vi "Handle State Value Table Change.vi"(7 "Routing Channel Page Controls":T1, 8 "error in (no error)":errorcluster, 9 "OldVal":T3[](array[typedef]), 10 "NewVal":T3[](array[typedef]), 11 "routing channel in":T2 format="%.0x") -> (0 "error out":errorcluster, 3 "routing channel out":T2 format="%.0x")   [LabVIEW 2017, in "Routing and Faulting System Explorer.lvlib"]
uses:
  <vilib>/NI Veristand/Custom Device API/Custom Device Item Ref.ctl
  State-Value Row.ctl
  Routing Channel Page Controls.ctl
  88e8a73d-5bf6-438f-825b-ec6305f3fa8d.vi
  Routing and Faulting System Explorer.lvlib
  Scripting/Routing and Faulting Scripting.lvlib
  <vilib>/NI Veristand/Custom Device API/Custom Device API.lvlib
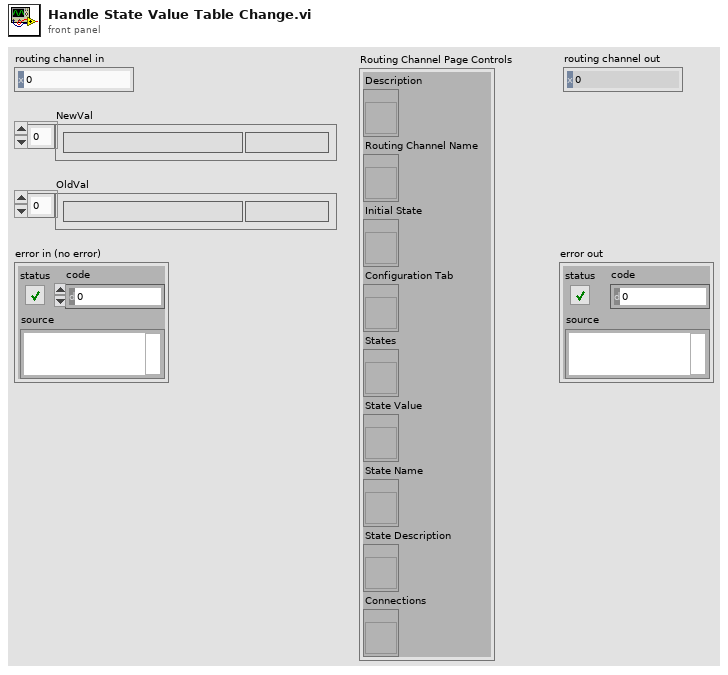
[diagram p1: front panel]
types:
  T1 = typedef "Routing and Faulting System Explorer.lvlib/Routing Channel Page Controls.ctl" = cluster{"Description":refnum<vi>, "Routing Channel Name":refnum<vi>, "Initial State":refnum<vi>, "Configuration Tab":refnum<vi>, "States":refnum<vi>, "State Value":refnum<vi>, "State Name":refnum<vi>, "State Description":refnum<vi>, "Connections":refnum<vi>}
  T2 = typedef "Custom Device API.lvlib/Custom Device Item Ref.ctl" = u64
  T3 = typedef "Routing and Faulting System Explorer.lvlib/State-Value Row.ctl" = cluster{"State":string, "State Value":string}
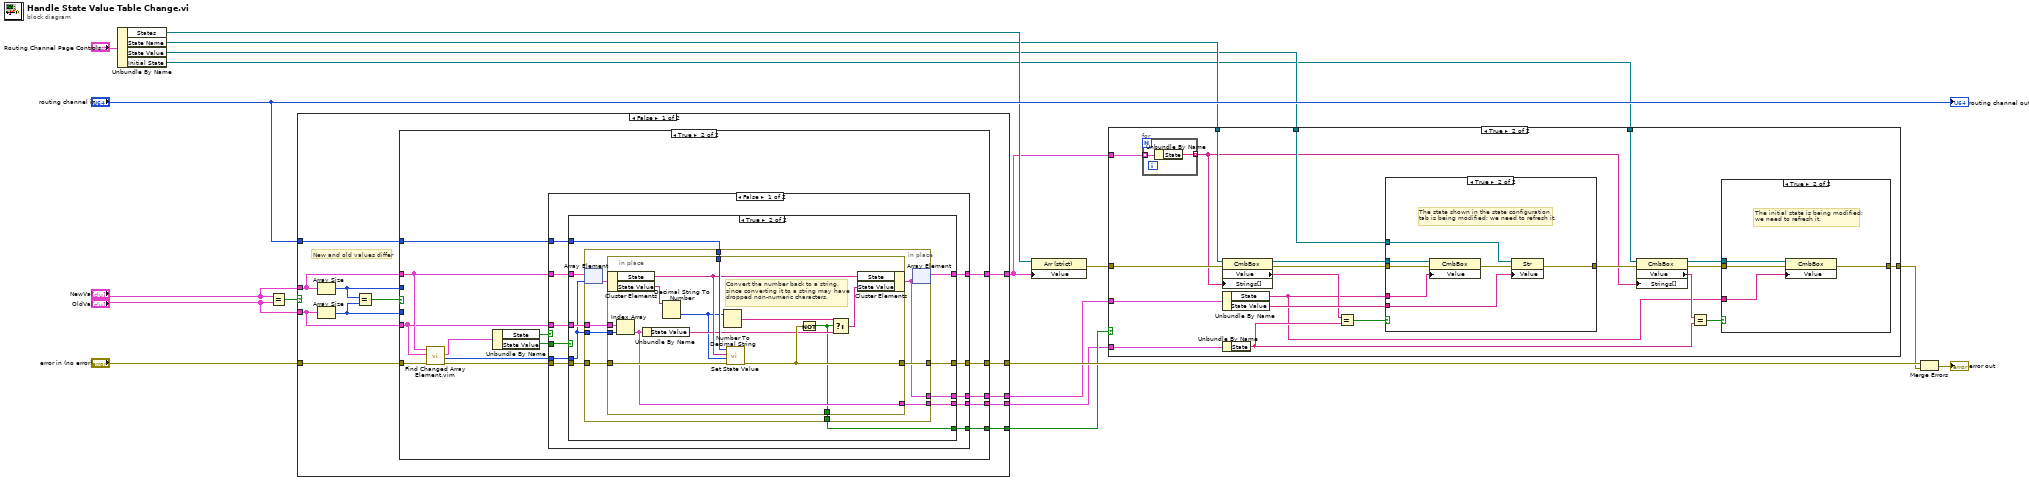
[diagram p0: block diagram]
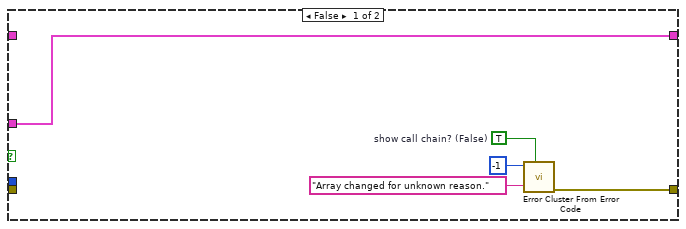
[diagram p3: hidden frame]
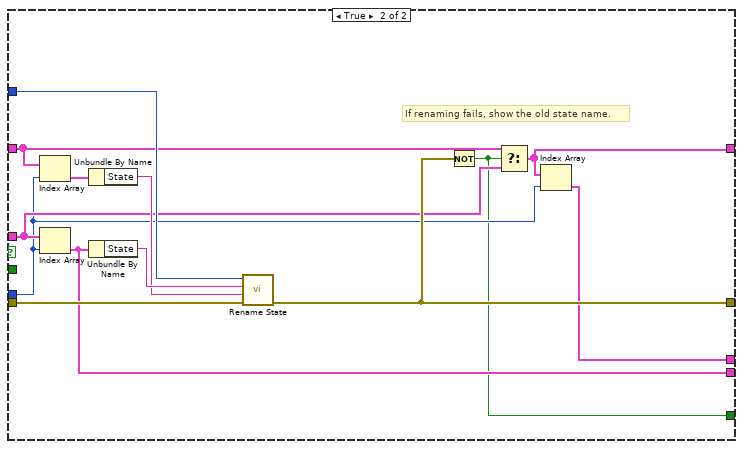
[diagram p4: hidden frame]
diagram:
  n1 = Unbundle By Name("Routing Channel Page Controls") -> ("States"=w10:refnum<vi>, "State Name"=w8:refnum<vi>, "State Value"=w4:refnum<vi>, "Initial State"=w1:refnum<vi>)
  n2 = Equal?(x="NewVal", y="OldVal") -> (x = y?=w13:bool)
  n3 = case shown="False" w13 {
    tunnel: "NewVal" -> [w27 w108]
    tunnel: "OldVal" -> [w26 _]
    tunnel: "routing channel in" -> [w25 _]
    tunnel: [w24 w109] -> w18
    tunnel: "error in (no error)" -> [w23 w109]
    tunnel: [w22 w108] -> w2
    tunnel: [w21 _] -> w7
    tunnel: [w20 _] -> w6
    tunnel: [w19 _] -> w5
    frame False {
      # "New and old values differ"
      n4 = Array Size(array=w27) -> (size(s)=w29:i32)
      n5 = Array Size(array=w26) -> (size(s)=w28:i32)
      n6 = Equal?(x=w29, y=w28) -> (x = y?=w30:bool)
      n7 = case shown="True" w30 {
        tunnel: w29 -> [_ _]
        tunnel: w28 -> [_ _]
        tunnel: w27 -> [_ w42]
        tunnel: w26 -> [w31 w37]
        tunnel: w25 -> [_ w44]
        tunnel: [w32 w41] -> w24
        tunnel: w23 -> [w32 w40]
        tunnel: [w31 w38] -> w22
        tunnel: [_ w35] -> w19
        tunnel: [_ w34] -> w20
        tunnel: [_ w33] -> w21
        frame False {
          # "This case can happen if items are inserted or removed from the array\nshortcut menu during runtime. This is a lot of extra code to handle,\nso the shortcut menu for the array on Endpoint Aliases Page.vi is\ncurrently disabled to prevent this code path.\nIf the shortcut menu is ever re-enabled, code for handling add/remove\nshould go in this case."
        }
        frame True {
          n8 = call "Find Changed Array Element.vim"("error in (no error)"=w40, "OldVal"=w37, "NewVal"=w42) -> ("error out"=w43:errorcluster, "Array Index"=w36:i32, "Element Changed"=w46:cluster{"State":bool, "State Value":bool})  [unwired: 6 in]
          n9 = Unbundle By Name(w46) -> ("State"=w45:bool, "State Value"=w39:bool)
          n10 = case shown="False" w45 {
            tunnel: w44 -> [w57 w107]
            tunnel: w43 -> [w54 w106]
            tunnel: w42 -> [w53 w101]
            tunnel: w37 -> [w50 w99]
            tunnel: [w55 w102] -> w41
            tunnel: w36 -> [w52 w97]
            tunnel: w39 -> [w56 _]
            tunnel: [w51 w100] -> w38
            tunnel: [w48 w98] -> w34
            tunnel: [w49 w96] -> w35
            tunnel: [w47 w95] -> w33
            frame False {
              n11 = case shown="True" w56 {
                tunnel: w57 -> [_ w70]
                tunnel: [w62 w71] -> w55
                tunnel: w54 -> [_ w72]
                tunnel: w53 -> [_ w69]
                tunnel: w52 -> [_ w66]
                tunnel: [w58 w68] -> w51
                tunnel: w50 -> [w58 w67]
                tunnel: [_ w65] -> w49
                tunnel: [_ w64] -> w48
                tunnel: [_ w63] -> w47
                frame False {
                  w59 = TRUE  # show call chain? (False)
                  n12 = call <vilib>:"Error Cluster From Error Code.vi"("show call chain? (False)"=w59, "error message (\"\")"="Array changed for unknown reason." ("error message (\"\")"), "error code (0)"=-1) -> ("error out"=w62:errorcluster)  [unwired: 6 in]
                }
                frame True {
                  n13 = in-place {
                    in-place-border: w72 -> [w81]
                    in-place-border: [w80] -> w71
                    in-place-border: w70 -> [w79]
                    in-place-border: w67 -> [w77]
                    in-place-border: w66 -> [w76]
                    in-place-border: [w75] -> w65
                    in-place-border: [w74] -> w64
                    in-place-border: [w73] -> w63
                    n14 = in-place-array #1(w69, w66) -> (w78:T3)
                    n15 = in-place {
                      in-place-border: w81 -> [w94]
                      in-place-border: [w93] -> w80
                      in-place-border: w79 -> [w92]
                      in-place-border: w77 -> [w88]
                      in-place-border: w76 -> [w87]
                      in-place-border: [w83] -> w74
                      in-place-border: [w82] -> w73
                      # "Convert the number back to a string,\nsince converting it to a string may have\ndropped non-numeric characters."
                      n16 = in-place-cluster #2(w78) -> ("State"=w89:string, "State Value"=w91:string)
                      n17 = Index Array(array=w88, index=w87) -> (element=w83:T3)
                      n18 = Unbundle By Name(w83) -> ("State Value"=w86:string)
                      n19 = Decimal String To Number(string=w91) -> (number=w85:i32)  [unwired: 2 in, 1 out]
                      n20 = Number To Decimal String(number=w85) -> (decimal integer string=w84:string)  [unwired: 1 in]
                      n21 = call "Set State Value.vi"("error in"=w94, "value"=w85, "state"=w89, "routing channel in"=w92) -> ("error out"=w93:errorcluster)  [unwired: 6 in, 1 out]
                      n22 = Not(x=w93) -> (.not. x?=w82:bool)
                      n23 = Select(t=w84, s=w82, f=w86) -> (s? t:f=w90:string)
                      n24 = in-place-cluster #2("State"=w89, "State Value"=w90) -> (w75:T3)
                    }
                    n25 = in-place-array #1(w75) -> (w68:T3[])  [unwired: 1 out]
                  }
                }
              }
            }
            frame True {
              # "If renaming fails, show the old state name."
              n26 = Index Array(array=w101, index=w97) -> (element=w105:T3)
              n27 = Index Array(array=w99, index=w97) -> (element=w98:T3)
              n28 = Unbundle By Name(w105) -> ("State"=w103:string)
              n29 = Unbundle By Name(w98) -> ("State"=w104:string)
              n30 = call "Rename State.vi"("error in"=w106, "new state"=w103, "state"=w104, "routing channel in"=w107) -> ("error out"=w102:errorcluster)  [unwired: 6 in, 1 out]
              n31 = Not(x=w102) -> (.not. x?=w95:bool)
              n32 = Select(t=w101, s=w95, f=w99) -> (s? t:f=w100:T3[])
              n33 = Index Array(array=w100, index=w97) -> (element=w96:T3)
            }
          }
        }
      }
    }
    frame True {
      # "New and old values are the same. Do nothing"
    }
  }
  n34 = property class="Arr (strict)"(reference=w10, "Value"=w2) -> (error out=w3:errorcluster)  [unwired: 1 in, 1 out]
  n35 = case shown="True" w7 {
    tunnel: [w110 w115] -> w9
    tunnel: w8 -> [_ w123]
    tunnel: w6 -> [_ w130]
    tunnel: w5 -> [_ w129]
    tunnel: w4 -> [_ w124]
    tunnel: w3 -> [w110 w128]
    tunnel: w2 -> [_ w127]
    tunnel: w1 -> [_ w121]
    frame False {
    }
    frame True {
      n36 = for {
        tunnel: w127 -> [w141] mode=indexing
        tunnel: [w140] -> w119 mode=indexing
        n37 = Unbundle By Name(w141) -> ("State"=w140:string)
      }
      n38 = property class="CmbBox"(reference=w123, error in=w128, "Strings[]"=w119) -> (reference out=w111:refnum<vi>, error out=w126:errorcluster, "Value"=w118:string)
      n39 = Unbundle By Name(w129) -> ("State"=w113:string, "State Value"=w122:string)
      n40 = Unbundle By Name(w130) -> ("State"=w117:string)
      n41 = Equal?(x=w118, y=w117) -> (x = y?=w125:bool)
      n42 = case shown="True" w125 {
        tunnel: [w132 w139] -> w131
        tunnel: w126 -> [w132 w138]
        tunnel: w124 -> [_ w137]
        tunnel: w113 -> [_ w135]
        tunnel: w122 -> [_ w134]
        tunnel: w111 -> [_ w133]
        frame False {
        }
        frame True {
          # "The state shown in the state configuration\ntab is being modified; we need to refresh it."
          n43 = property class="CmbBox"(reference=w133, error in=w138, "Value"=w135) -> (error out=w136:errorcluster)  [unwired: 1 out]
          n44 = property class="Str"(reference=w137, error in=w136, "Value"=w134) -> (error out=w139:errorcluster)  [unwired: 1 out]
        }
      }
      n45 = property class="CmbBox"(reference=w121, error in=w131, "Strings[]"=w119) -> (reference out=w112:refnum<vi>, error out=w116:errorcluster, "Value"=w120:string)
      n46 = Equal?(x=w120, y=w117) -> (x = y?=w114:bool)
      n47 = case shown="True" w114 {
        tunnel: w116 -> [w142 w146]
        tunnel: [w142 w145] -> w115
        tunnel: w113 -> [_ w144]
        tunnel: w112 -> [_ w143]
        frame False {
        }
        frame True {
          # "The initial state is being modified;\nwe need to refresh it."
          n48 = property class="CmbBox"(reference=w143, error in=w146, "Value"=w144) -> (error out=w145:errorcluster)  [unwired: 1 out]
        }
      }
    }
  }
  n49 = Merge Errors(w18, w9) -> (→"error out":errorcluster)
  "routing channel out" <- "routing channel in"
